vi "Main - Decrypt (SubVI).vi"(10 "Base64 String":string) -> (3 "String":string)   [LabVIEW 2019]
panel:
  out "error out":errorcluster
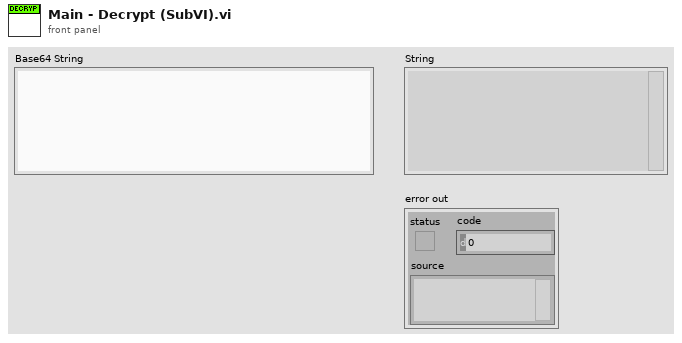
[diagram p1: front panel]
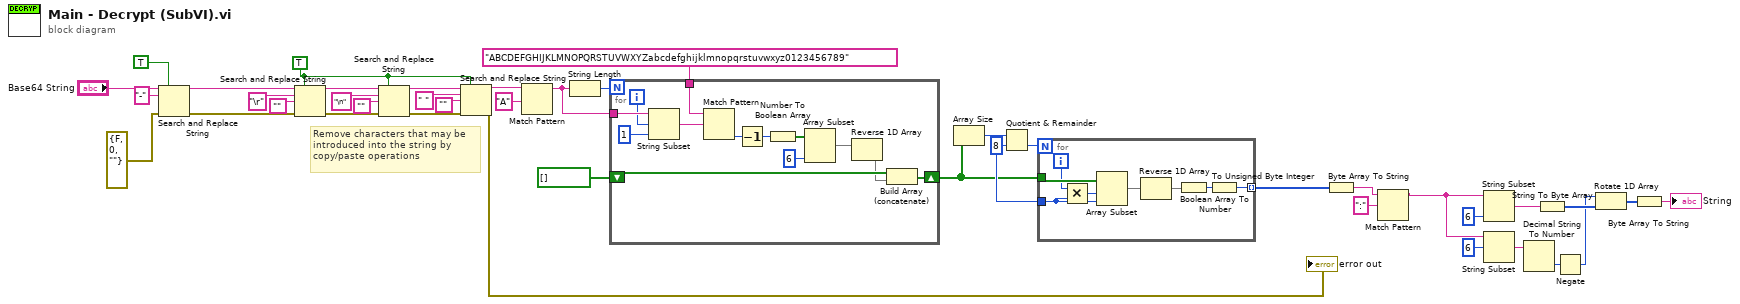
[diagram p0: block diagram]
diagram:
  w41 = TRUE ("replace all? (F)")
  w28 = 8 ("y")
  # "Remove characters that may be\nintroduced into the string by\ncopy/paste operations"
  n1 = Search and Replace String(replace all?=TRUE ("replace all? (F)"), input string="Base64 String", search string="-", error in=errorcluster {"status"=FALSE, "code"=0, "source"=""} ("error in (no error)")) -> (result string=w5:string, error out=w3:errorcluster)  [unwired: 4 in, 2 out]
  n2 = Search and Replace String(replace all?=w41, input string=w5, search string="\r" ("replace string (\"\")"), replace string="", error in=w3) -> (result string=w32:string, error out=w34:errorcluster)  [unwired: 5 out]
  n3 = Search and Replace String(replace all?=w41, input string=w32, search string="\n" ("replace string (\"\")"), replace string="", error in=w34) -> (result string=w37:string, error out=w38:errorcluster)  [unwired: 5 out]
  n4 = Search and Replace String(replace all?=w41, input string=w37, search string=" " ("replace string (\"\")"), replace string="", error in=w38) -> (result string=w40:string, error out=→"error out":errorcluster)  [unwired: 5 out]
  n5 = Match Pattern(string=w40, regular expression="A") -> (before substring=w23:string)  [unwired: 4 out]
  n6 = String Length(string=w23) -> (length=w20:i32)
  n7 = for {
    N: w20 -> [_]
    tunnel: w23 -> [w54]
    tunnel: "ABCDEFGHIJKLMNOPQRSTUVWXYZabcdefghijklmnopqrstuvwxyz0123456789" -> [w51]
    shift-right: [w44] -> w27
    shift-left: bool[] [] -> [w43]
    i -> [w52]
    n8 = String Subset(string=w54, offset (0)=w52, length (rest)=1 ("length (rest)")) -> (substring=w50:string)
    n9 = Match Pattern(string=w51, regular expression=w50) -> (offset past match=w49:i32)  [unwired: 1 in, 3 out]
    n10 = Decrement(x=w49) -> (x-1=w48:i32)
    n11 = Number To Boolean Array(number=w48) -> (Boolean array=w47:bool[])
    n12 = Array Subset(array=w47, length=6) -> (w45:bool[])  [unwired: 1 in]
    n13 = Reverse 1D Array(array=w45) -> (reversed array=w42:bool[])
    n14 = Build Array (concatenate)(w43, w42) -> (w44:bool[])
  }
  n15 = Array Size(array=w27) -> (size(s)=w25:i32)
  n16 = Quotient & Remainder(x=w25, y=w28) -> (floor(x/y)=w26:i32)  [unwired: 1 out]
  n17 = for {
    N: w26 -> [_]
    tunnel: w27 -> [w62]
    tunnel: w28 -> [w61]
    tunnel: [w57] -> w2 mode=indexing
    i -> [w60]
    n18 = Multiply(x=w60, y=w61) -> (x*y=w55:i32)
    n19 = Array Subset(array=w62, index=w55, length=w61) -> (w59:bool[])
    n20 = Reverse 1D Array(array=w59) -> (reversed array=w56:bool[])
    n21 = Boolean Array To Number(Boolean array=w56) -> (number=w58:u32)
    n22 = To Unsigned Byte Integer(number=w58) -> (unsigned 8bit integer=w57:u8)
  }
  n23 = Byte Array To String(unsigned byte array=w2) -> (string=w10:string)
  n24 = Match Pattern(string=w10, regular expression=":") -> (before substring=w11:string)  [unwired: 1 in, 3 out]
  n25 = String Subset(string=w11, length (rest)=6 ("length (rest)")) -> (substring=w17:string)  [unwired: 1 in]
  n26 = String Subset(string=w11, offset (0)=6) -> (substring=w15:string)  [unwired: 1 in]
  n27 = Decimal String To Number(string=w15) -> (number=w14:i32)  [unwired: 2 in, 1 out]
  n28 = String To Byte Array(string=w17) -> (unsigned byte array=w16:u8[])
  n29 = Negate(x=w14) -> (-x=w1:i32)
  n30 = Rotate 1D Array(1:w16, 2:w1) -> (0:w13:u8[])
  n31 = Byte Array To String(unsigned byte array=w13) -> (string=→"String":string)
